vi "GetEventStreamByIdAndCategory.vi"(8 "error in":errorcluster, 10 "Category":string, 11 "ID":string) -> (0 "error out":errorcluster, 2 "Event Stream Out":refnum<user-event>, 3 "Event Registration Refnum out":refnum<event-registration>)   [LabVIEW 2017]
uses:
  Types/SystemEventDataStruct.ctl
  Globals/globals.vi
panel:
  out "StreamID":string
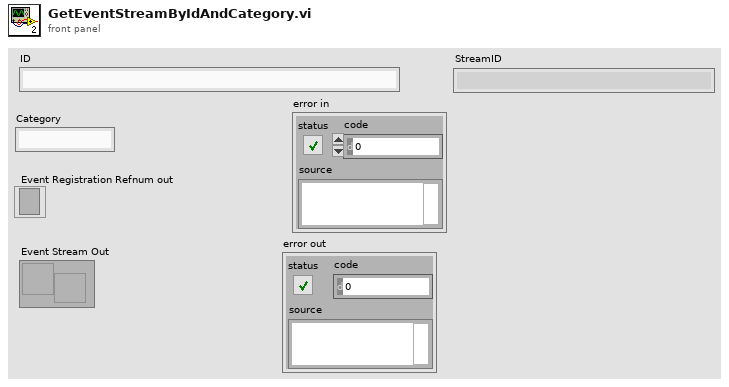
[diagram p1: front panel]
types:
  T1 = cluster{"Event Register":refnum<event-registration>, "Event Stream":refnum<user-event>}
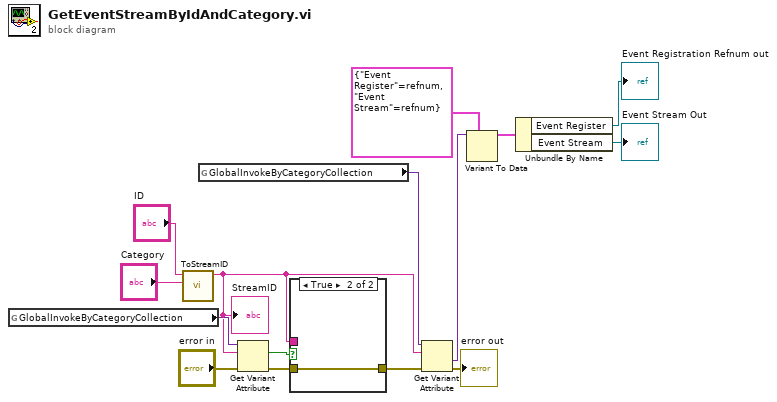
[diagram p0: block diagram]
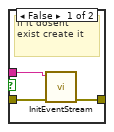
[diagram p2: hidden frame]
diagram:
  n1 = global read "globals.vi" "GlobalInvokeByCategoryCollection"() -> (w9:variant)
  n2 = call "ToStreamID.vi"("Category"="Category", "ID in"="ID") -> ("ID out"=w7:string)  [unwired: 9 in]
  "StreamID" <- w7
  n3 = global read "globals.vi" "GlobalInvokeByCategoryCollection"() -> (w1:variant)
  n4 = Get Variant Attribute(Variant=w9, name=w7, error in="error in") -> (found=w8:bool, error out=w4:errorcluster)  [unwired: 1 in, 2 out]
  n5 = case shown="True" w8 {
    tunnel: w7 -> [w18 _]
    tunnel: w4 -> [w17 w19]
    tunnel: [w16 w19] -> w3
    frame False {
      # "If it dosent\nexist create it"
      n6 = call "InitEventStream.vi"("error in"=w17, "SteamID"=w18) -> ("error out"=w16:errorcluster)  [unwired: 8 in, 1 out]
    }
    frame True {
    }
  }
  n7 = Get Variant Attribute(Variant=w1, name=w7, error in=w3) -> (value=w6:variant, error out=→"error out":errorcluster)  [unwired: 1 in, 2 out]
  n8 = Variant To Data(type=T1 {"Event Register"=refnum, "Event Stream"=refnum}, Variant=w6) -> (data=w10:T1)  [unwired: 1 in, 1 out]
  n9 = Unbundle By Name(w10) -> ("Event Register"=→"Event Registration Refnum out":refnum<event-registration>, "Event Stream"=→"Event Stream Out":refnum<user-event>)
